vi "LEBITVacuum.SetSafeLL.vi"(0 "i ref in":refnum<vi>, 1 "Set Safety":i16, 2 "i attribute in":T1={"setValuePLC"=[], "nickNames"=[], "setValuePLCServiceID"=[], "monValuePLC"=[], "SetValueServiceID"=[], "MonValueServiceID"=[], "SetValue"=[], "AllPLCValues"=[], "CondSpecial2DArray"=[], "CondSpecialIndex"=[], "ReasonForLocking"="", "ReasonForLockingID"=0, "enableValuePLC"=[], "OverwriteCloseSafetyPLC"=[], "OverwriteOpenSafetyPLC"=[], "OverwriteCloseSafetyPLCServiceID"=[], "OverwriteOpenSafetyPLCServiceID"=[], "MKS Address Array"=[], "MKS MeasurementServiceID"=[], "MKS Measurement"=[], "CRYO Measurement"=[], "CRYO MeasurementServiceID"=[], "Special"=[], "Start Date"="", "MKS VISA resource"="COM13", "CRYO VISA resource"="COM13"}, 3 "SetValue":i16, 4 "index of element":i32, 5 "error IO":errorcluster) -> (14 "i ref out":refnum<vi>, 15 "i attribute out":T1={"setValuePLC"=[], "nickNames"=[], "setValuePLCServiceID"=[], "monValuePLC"=[], "SetValueServiceID"=[], "MonValueServiceID"=[], "SetValue"=[], "AllPLCValues"=[], "CondSpecial2DArray"=[], "CondSpecialIndex"=[], "ReasonForLocking"="", "ReasonForLockingID"=0, "enableValuePLC"=[], "OverwriteCloseSafetyPLC"=[], "OverwriteOpenSafetyPLC"=[], "OverwriteCloseSafetyPLCServiceID"=[], "OverwriteOpenSafetyPLCServiceID"=[], "MKS Address Array"=[], "MKS MeasurementServiceID"=[], "MKS Measurement"=[], "CRYO Measurement"=[], "CRYO MeasurementServiceID"=[], "Special"=[], "Start Date"="", "MKS VISA resource"="COM13", "CRYO VISA resource"="COM13"}, 19 "error out":errorcluster)   [LabVIEW 2014, in "LEBITVacuum.lvlib"]
uses:
  LEBITVacuum.lvlib
  LEBITVacuum.i attribute.ctl
  CSlibraries-extern/DimLVEvent/LVDimInterface/LVDimInterface.lvlib
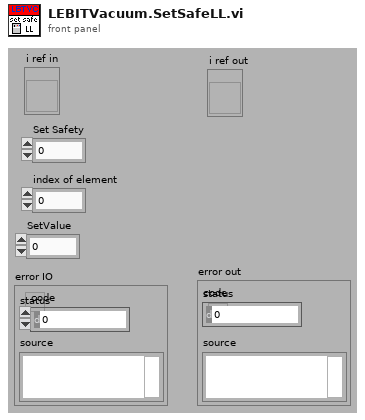
[diagram p1: front panel]
types:
  T1 = typedef "LEBITVacuum.lvlib/LEBITVacuum.i attribute.ctl" = cluster{"setValuePLC":string[], "nickNames":string[], "setValuePLCServiceID":i32[], "monValuePLC":string[], "SetValueServiceID":i32[], "MonValueServiceID":i32[], "SetValue":i16[], "AllPLCValues":string[], "CondSpecial2DArray":string[][], "CondSpecialIndex":i32[], "ReasonForLocking":string, "ReasonForLockingID":i32, "enableValuePLC":string[], "OverwriteCloseSafetyPLC":string[], "OverwriteOpenSafetyPLC":string[], "OverwriteCloseSafetyPLCServiceID":i32[], "OverwriteOpenSafetyPLCServiceID":i32[], "MKS Address Array":i32[][], "MKS MeasurementServiceID":i32[], "MKS Measurement":string[], "CRYO Measurement":string[][], "CRYO MeasurementServiceID":i32[], "Special":string[], "Start Date":string, "MKS VISA resource":refnum<visa-resource-name>, "CRYO VISA resource":refnum<visa-resource-name>}
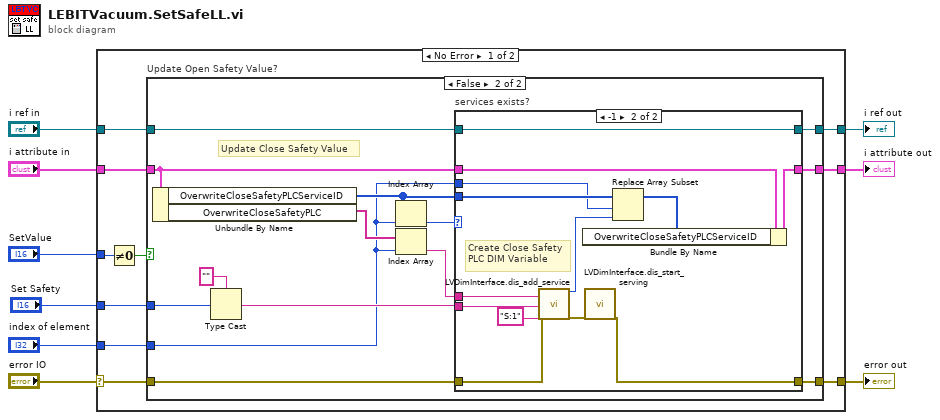
[diagram p0: block diagram]
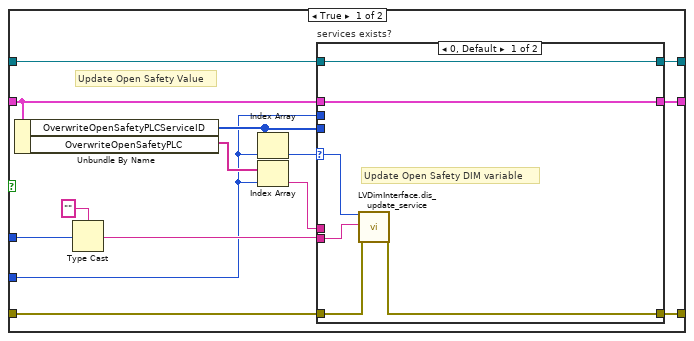
[diagram p2: hidden frame]
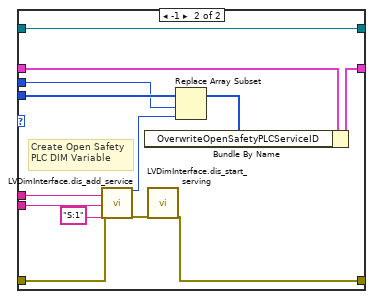
[diagram p3: hidden frame]
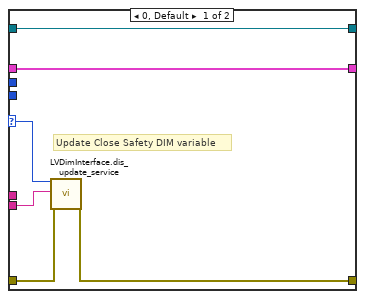
[diagram p4: hidden frame]
diagram:
  n1 = case shown="No Error" "error IO" {
    selector: "error IO" -> [w15 w86]
    tunnel: "index of element" -> [w13 _]
    tunnel: "i attribute in" -> [w14 w87]
    tunnel: [w19 w87] -> w7
    tunnel: [w18 w86] -> w6
    tunnel: [w17 w88] -> w5
    tunnel: "i ref in" -> [w16 w88]
    tunnel: "SetValue" -> [w11 _]
    tunnel: "Set Safety" -> [w12 _]
    frame No Error {
      n2 = Not Equal To 0?(x=w11) -> (x != 0?=w10:bool)
      n3 = case "Update Open Safety Value?" shown="False" w10 {
        tunnel: [w33 w66] -> w19
        tunnel: [w32 w65] -> w18
        tunnel: [w31 w64] -> w17
        tunnel: w16 -> [w30 w63]
        tunnel: w15 -> [w20 w53]
        tunnel: w14 -> [w23 w56]
        tunnel: w13 -> [w22 w55]
        tunnel: w12 -> [w21 w54]
        frame True {
          # "Update Open Safety Value"
          n4 = Unbundle By Name(w23) -> ("OverwriteOpenSafetyPLCServiceID"=w27:i32[], "OverwriteOpenSafetyPLC"=w24:string[])
          n5 = Type Cast(type="", x=w21) -> (*(type *) &x=w25:string)
          n6 = Index Array(array=w27, index=w22) -> (element=w28:i32)
          n7 = Index Array(array=w24, index=w22) -> (element=w29:string)
          n8 = case "services exists?" shown="0, Default" w28 {
            selector: w28 -> [w39 _]
            tunnel: w25 -> [w38 w40]
            tunnel: w29 -> [_ w41]
            tunnel: w30 -> [w37 w47]
            tunnel: [w37 w47] -> w31
            tunnel: w20 -> [w35 w45]
            tunnel: w27 -> [_ w52]
            tunnel: [w34 w43] -> w32
            tunnel: w22 -> [_ w51]
            tunnel: w23 -> [w36 w48]
            tunnel: [w36 w46] -> w33
            frame 0, Default {
              # "Update Open Safety DIM variable"
              n9 = call "LVDimInterface.dis_update_service.vi"("my_serviceID"=w39, "data"=w38, "error in (no error)"=w35) -> ("error out"=w34:errorcluster)  [unwired: 14 in, 2 out]
            }
            frame -1 {
              # "Create Open Safety\nPLC DIM Variable"
              n10 = call "LVDimInterface.dis_add_service.vi"("serviceName"=w41, "typeDescriptor"="S:1", "data"=w40, "error in (no error)"=w45) -> ("my_serviceID"=w50:i32, "error out"=w44:errorcluster)  [unwired: 14 in]
              n11 = call "LVDimInterface.dis_start_serving.vi"("error in (no error)"=w44) -> ("error out"=w43:errorcluster)  [unwired: 17 in, 1 out]
              n12 = Replace Array Subset(array=w52, new element=w50, index=w51) -> (w49:i32[])
              n13 = Bundle By Name(cluster=w48, "OverwriteOpenSafetyPLCServiceID"=w49) -> (w46:T1)
            }
          }
        }
        frame False {
          # "Update Close Safety Value"
          n14 = Unbundle By Name(w56) -> ("OverwriteCloseSafetyPLCServiceID"=w60:i32[], "OverwriteCloseSafetyPLC"=w57:string[])
          n15 = Type Cast(type="", x=w54) -> (*(type *) &x=w58:string)
          n16 = Index Array(array=w60, index=w55) -> (element=w61:i32)
          n17 = Index Array(array=w57, index=w55) -> (element=w62:string)
          n18 = case "services exists?" shown="-1" w61 {
            selector: w61 -> [w72 _]
            tunnel: w58 -> [w71 w73]
            tunnel: w62 -> [_ w74]
            tunnel: w63 -> [w70 w80]
            tunnel: [w70 w80] -> w64
            tunnel: w53 -> [w68 w78]
            tunnel: w60 -> [_ w85]
            tunnel: [w67 w76] -> w65
            tunnel: w55 -> [_ w84]
            tunnel: w56 -> [w69 w81]
            tunnel: [w69 w79] -> w66
            frame 0, Default {
              # "Update Close Safety DIM variable"
              n19 = call "LVDimInterface.dis_update_service.vi"("my_serviceID"=w72, "data"=w71, "error in (no error)"=w68) -> ("error out"=w67:errorcluster)  [unwired: 14 in, 2 out]
            }
            frame -1 {
              # "Create Close Safety\nPLC DIM Variable"
              n20 = call "LVDimInterface.dis_add_service.vi"("serviceName"=w74, "typeDescriptor"="S:1", "data"=w73, "error in (no error)"=w78) -> ("my_serviceID"=w83:i32, "error out"=w77:errorcluster)  [unwired: 14 in]
              n21 = call "LVDimInterface.dis_start_serving.vi"("error in (no error)"=w77) -> ("error out"=w76:errorcluster)  [unwired: 17 in, 1 out]
              n22 = Replace Array Subset(array=w85, new element=w83, index=w84) -> (w82:i32[])
              n23 = Bundle By Name(cluster=w81, "OverwriteCloseSafetyPLCServiceID"=w82) -> (w79:T1)
            }
          }
        }
      }
    }
    frame Error {
    }
  }
  "i attribute out" <- w7
  "error out" <- w6
  "i ref out" <- w5
